vi "CVT2_GenTags.vi"(11 "Tags per type":i32) -> (0 "names":string[](array[string]), 1 "Values":i32[](array[numeric]), 2 "Init data":T1, 3 "Tags per type out":i32)   [LabVIEW 2013, in "UnitTests.lvlib"]
uses:
  UnitTests.lvlib
  <vilib>/NI/Current Value Table/Type Defs/File Format.ctl
  <vilib>/NI/Current Value Table/Type Defs/Single Tag.ctl
  <vilib>/NI/Current Value Table/Type Defs/Data Types.ctl
  <vilib>/NI/Current Value Table/Type Defs/Tag Grouping set.ctl
  <vilib>/NI/Current Value Table/Current Value Table.lvlib
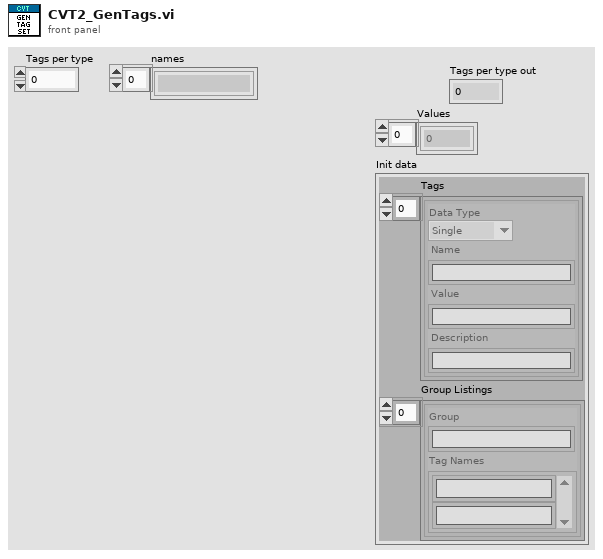
[diagram p1: front panel]
types:
  T1 = typedef "Current Value Table.lvlib/File Format.ctl" = cluster{"Tags":T2[], "Group Listings":T4[]}
  T2 = typedef "Current Value Table.lvlib/Single Tag.ctl" = cluster{"Data Type":T3, "Name":string, "Value":string, "Description":string}
  T3 = typedef "Current Value Table.lvlib/Data Types.ctl" = enum16{"Double", "Single", "I64", "I32", "I16", "I8", "U64", "U32", "U16", "U8", "String", "Boolean", "Array of U8", "Array of U16", "Array of U32", "Array of U64", "Array of I64", "Array of I32", "Array of I16", "Array of I8", "Array of Double", "Array of Single", "Array of Boolean", "Array of String"}
  T4 = typedef "Current Value Table.lvlib/Tag Grouping set.ctl" = cluster{"Group":string, "Tag Names":string[]}
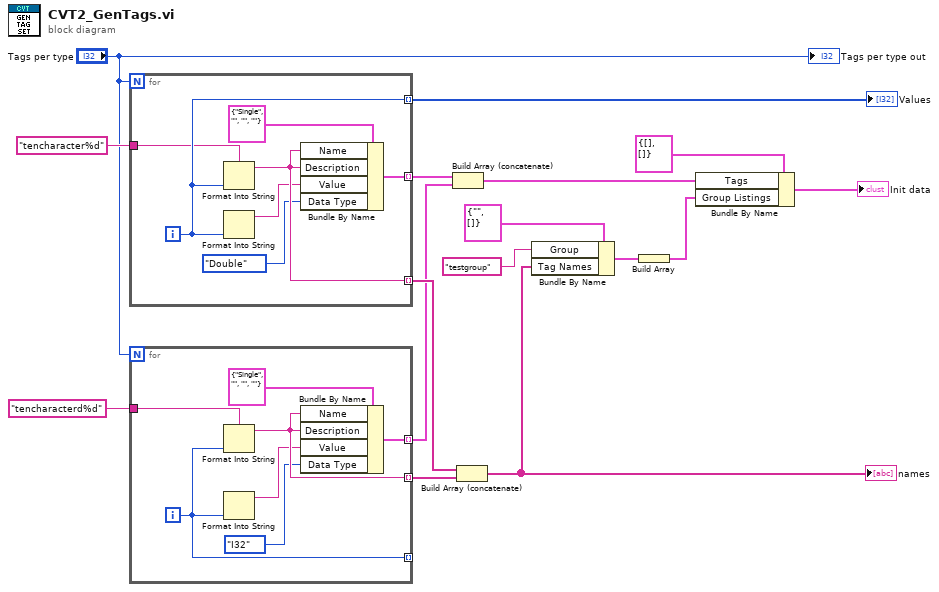
[diagram p0: block diagram]
diagram:
  n1 = for {
    N: "Tags per type" -> [_]
    tunnel: [w23] -> w5 mode=indexing
    tunnel: [w22] -> w9 mode=indexing
    tunnel: [w20] -> w14 mode=indexing
    tunnel: "tencharacter%d" ("format string") -> [w19]
    i -> [w20]
    n2 = Format Into String(format string=w19, w20) -> (resulting string=w22:string)  [unwired: 2 in, 1 out]
    n3 = Format Into String(w20) -> (resulting string=w21:string)  [unwired: 3 in, 1 out]
    n4 = Bundle By Name(cluster=T2 {"Data Type"=enum."Single", "Name"="", "Value"="", "Description"=""} ("Tag"), "Name"=w22, "Description"=w22, "Value"=w21, "Data Type"=Data_Types."Double") -> (w23:T2)
  }
  "Values" <- w14
  n5 = for {
    N: "Tags per type" -> [_]
    tunnel: [w30] -> w4 mode=indexing
    tunnel: [w29] -> w10 mode=indexing
    tunnel: [w27] -> _ mode=indexing
    tunnel: "tencharacterd%d" ("format string") -> [w26]
    i -> [w27]
    n6 = Format Into String(format string=w26, w27) -> (resulting string=w29:string)  [unwired: 2 in, 1 out]
    n7 = Format Into String(w27) -> (resulting string=w28:string)  [unwired: 3 in, 1 out]
    n8 = Bundle By Name(cluster=T2 {"Data Type"=enum."Single", "Name"="", "Value"="", "Description"=""} ("Tag"), "Name"=w29, "Description"=w29, "Value"=w28, "Data Type"=Data_Types."I32") -> (w30:T2)
  }
  n9 = Build Array (concatenate)(w5, w4) -> (w3:T2[])
  n10 = Build Array (concatenate)(w9, w10) -> (w8:string[])
  "names" <- w8
  n11 = Bundle By Name(cluster=T4 {"Group"="", "Tag Names"=[]} ("Tag Grouping"), "Group"="testgroup", "Tag Names"=w8) -> (w15:T4)
  n12 = Build Array(w15) -> (w12:T4[])
  n13 = Bundle By Name(cluster=T1 {"Tags"=[], "Group Listings"=[]} ("Tag Set"), "Tags"=w3, "Group Listings"=w12) -> (→"Init data":T1)
  "Tags per type out" <- "Tags per type"
